vi "stdout.vi"(4 "error in (no error)":errorcluster, 7 "data":string) -> (0 "error out":errorcluster, 3 "bytes written":i32)   [LabVIEW 2014]
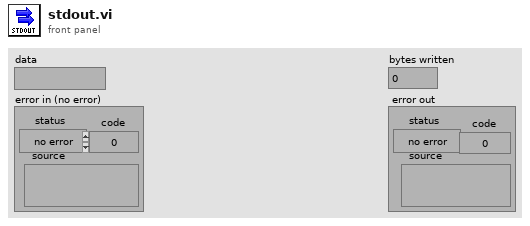
[diagram p1: front panel]
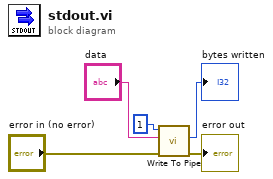
[diagram p0: block diagram]
diagram:
  n1 = call <vilib>:"Write To Pipe.vi"("error in (no error)"="error in (no error)", "data"="data", "file descriptor"=1) -> ("error out"=→"error out":errorcluster, "bytes written"=→"bytes written":i32)  [unwired: 2 in, 1 out]
